vi "Example SubVI.vi"() -> ()   [LabVIEW 2025]
panel:
  out "Seconds Alive":dbl format="%.1g"
  # "Example SubVI UI Running on cRIO"
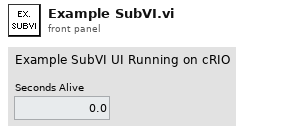
[diagram p1: front panel]
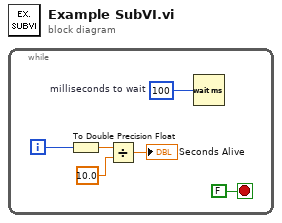
[diagram p0: block diagram]
diagram:
  n1 = while {
    i -> [w3]
    stop <- FALSE stop-if-true
    w5 = u32 100  # milliseconds to wait
    n2 = To Double Precision Float(number=w3) -> (double precision float=w2:dbl)
    n3 = Divide(x=w2, y=10.0) -> (x/y=→"Seconds Alive":dbl)
    n4 = Wait (ms)(milliseconds to wait=w5) -> ()  [unwired: 1 out]
  }
